vi "Initialize Pump.vi"(8 "error in (no error)":errorcluster, 11 "Application in":refnum<class "Application.lvclass">) -> (0 "error out":errorcluster, 3 "Application out":refnum<class "Application.lvclass">)   [LabVIEW 2018, in "Application.lvlib" / "Application.lvclass"]
uses:
  Application.lvclass
  C:/Program Files/National Instruments/LabVIEW 2018/vi.lib/ActorFramework/Actor/Actor.lvclass
  Application.lvclass/Application.ctl
  Hardware/cetoni/cetoni.lvclass
  <vilib>/ActorFramework/Actor/Actor.lvclass
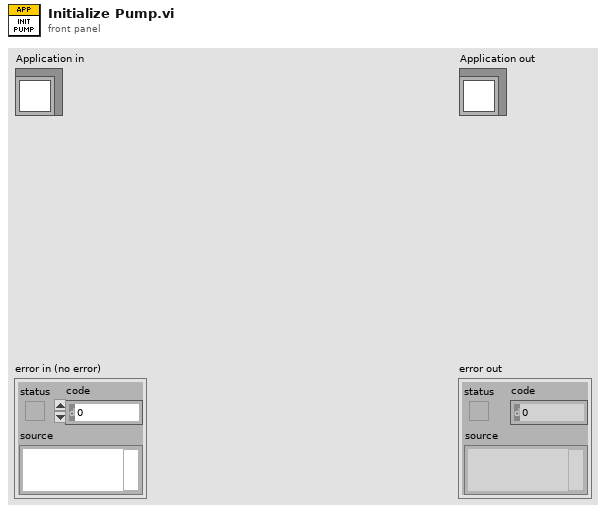
[diagram p1: front panel]
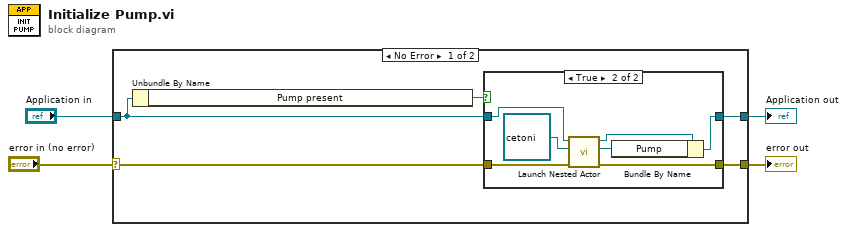
[diagram p0: block diagram]
diagram:
  n1 = case shown="No Error" "error in (no error)" {
    selector: "error in (no error)" -> [w6 w20]
    tunnel: [w7 w20] -> w3
    tunnel: [w8 w19] -> w1
    tunnel: "Application in" -> [w9 w19]
    frame No Error {
      n2 = Unbundle By Name(w9) -> ("Pump present"=w5:bool)
      n3 = case shown="True" w5 {
        tunnel: w9 -> [w10 w16]
        tunnel: [w10 w15] -> w8
        tunnel: [w11 w14] -> w7
        tunnel: w6 -> [w11 w13]
        frame False {
        }
        frame True {
          n4 = call <vilib>:"Launch Nested Actor.vi"("error in (no error)"=w13, "Nested Actor"=refnum<class "cetoni.lvclass"> refnum ("PHD Ultra.lvlib:PHD Ultra.lvclass"), "Caller Actor in"=w16) -> ("error out"=w14:errorcluster, "Nested Actor's Enqueuer"=w17:refnum<class "Message Enqueuer.lvclass">, "Caller Actor out"=w18:refnum<class "Application.lvclass">)  [unwired: 6 in]
          n5 = Bundle By Name(cluster=w18, "Pump"=w17) -> (w15:refnum<class "Application.lvclass">)
        }
      }
    }
    frame Error {
    }
  }
  "error out" <- w3
  "Application out" <- w1
